vi "read-pressure.vi"(8 "error in":errorcluster, 11 "Modbus instance in":refnum<class "Modbus Master.lvclass">) -> (0 "error out":errorcluster, 1 "Pirani":sgl, 2 "Ion Gauge":sgl, 3 "Modbus instance out":refnum<class "Modbus Master.lvclass">)   [LabVIEW 2016]
uses:
  <vilib>/NI/Modbus Library/API/Master/Modbus Master.lvclass
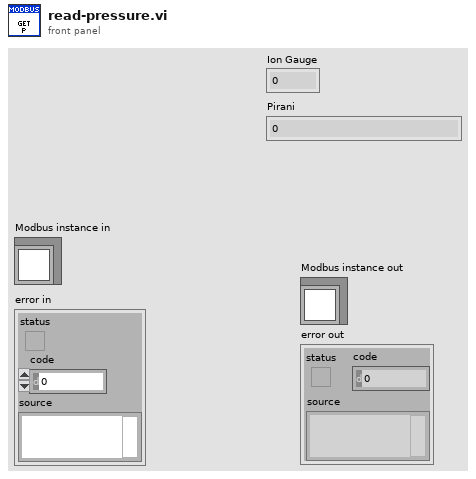
[diagram p1: front panel]
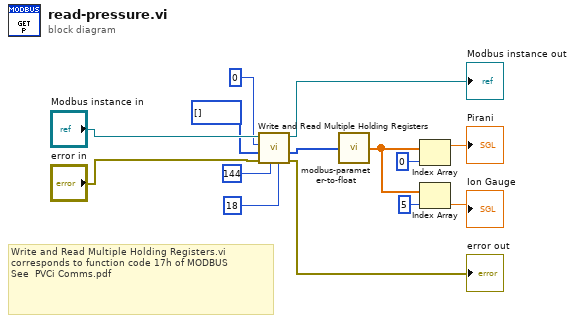
[diagram p0: block diagram]
diagram:
  # "Write and Read Multiple Holding Registers.vi corresponds to function code 17h of MODBUS\nSee  PVCi Comms.pdf"
  n1 = call-dynamic "Write and Read Multiple Holding Registers.vi"("read count"=u16 18, "read starting address"=u16 144, "error in"="error in", "write values"=u16[] [], "write starting address"=u16 0, "Modbus instance in"="Modbus instance in") -> ("error out"=→"error out":errorcluster, "read values"=w14:u16[], "Modbus instance out"=→"Modbus instance out":refnum<class "Modbus Master.lvclass">)  [unwired: 3 in]
  n2 = call "modbus-parameter-to-float.vi"("MODBUS parameter"=w14) -> ("float"=w9:sgl[])
  n3 = Index Array(array=w9, index=0) -> (element=→"Pirani":sgl)
  n4 = Index Array(array=w9, index=5) -> (element=→"Ion Gauge":sgl)
